vi "Initialize Connection with CD.vi"(8 "error in (no error)":errorcluster, 10 "TCP Service":string, 11 "IP Address":string) -> (0 "error out":errorcluster, 3 "Connection Info Out":T1)   [LabVIEW 2015, in "Instrument CD Host API.lvlib"]
uses:
  Instrument CD Host API.lvlib
  <vilib>/NI/STM/compatibility/stm_TCP Connection Info.ctl
  <vilib>/NI/STM/compatibility/stm_MetaDataElement.ctl
  <vilib>/NI/STM/compatibility/STM Write Meta Data (TCP Ref).vi
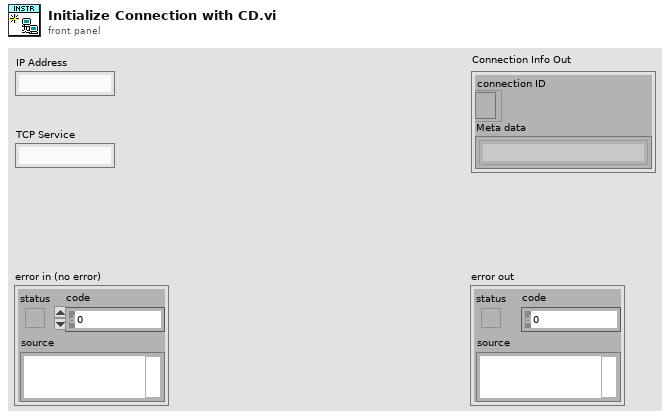
[diagram p1: front panel]
types:
  T1 = typedef "stm_TCP Connection Info.ctl" = cluster{"connection ID":refnum<k5>, "Meta data":T2[]}
  T2 = typedef "stm_MetaDataElement.ctl" = string
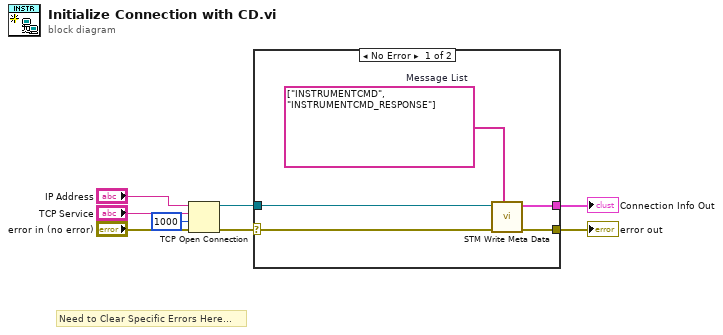
[diagram p0: block diagram]
diagram:
  # "Need to Clear Specific Errors Here..."
  n1 = TCP Open Connection(address="IP Address", remote port or service name="TCP Service", timeout ms (60000)=1000, error in (no error)="error in (no error)") -> (connection ID=w8:refnum<k5>, error out=w7:errorcluster)  [unwired: 1 in]
  n2 = case shown="No Error" w7 {
    selector: w7 -> [w10 w14]
    tunnel: w8 -> [w12 _]
    tunnel: [w11 w14] -> w1
    tunnel: [w9 _] -> w5
    frame No Error {
      w13 = string[] ["INSTRUMENTCMD", "INSTRUMENTCMD_RESPONSE"]  # Message List
      n3 = call-poly <vilib>:"STM Write Meta Data.vi"("Meta data"=w13, "error in"=w10, "connection ID"=w12) -> ("error out"=w11:errorcluster, "Connection Info Out"=w9:T1)  [unwired: 7 in]
    }
    frame Error {
    }
  }
  "error out" <- w1
  "Connection Info Out" <- w5
